vi "asdasd.vi"() -> ()   [LabVIEW 2018]
uses:
  <vilib>/userdefined/High Color/IMAQdx.ctl
  <vilib>/vision/Image Controls.llb/IMAQ Image.ctl
  <vilib>/vision/driver/NI_Vision_Acquisition_Software.lvlib
  <resource>/objmgr/imaqdx.rc
panel:
  in  "VideoMode":u32
  out "Image":T1(plugin-control)
  out "selected path":path caption="선택된 경로"
  out "Image Out":T1
  in  "Session In":T2
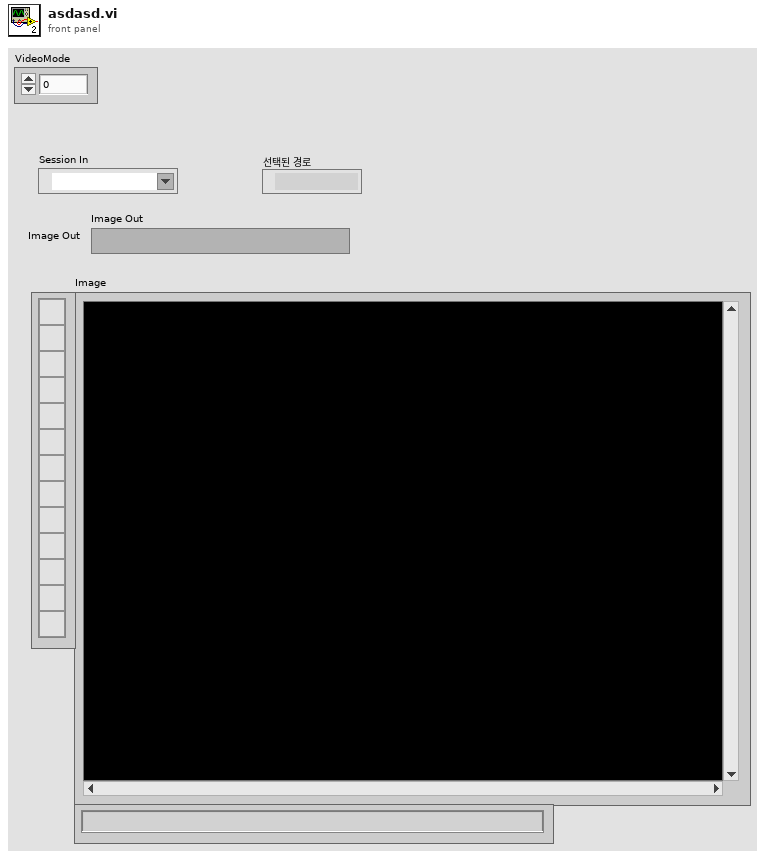
[diagram p1: front panel]
types:
  T1 = typedef "IMAQ Image.ctl" = refnum<image>
  T2 = typedef "IMAQdx.ctl" = refnum<k21>
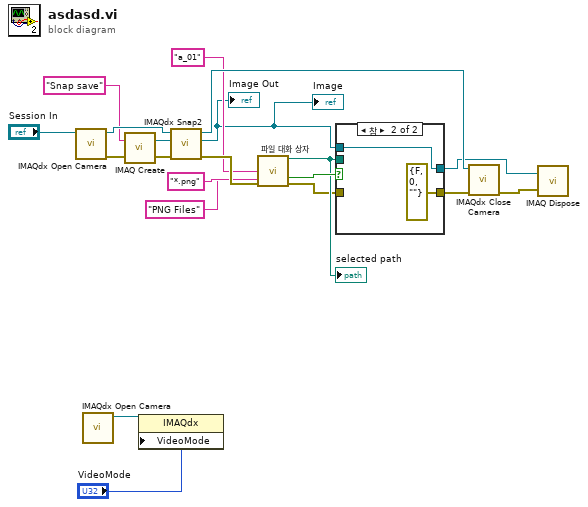
[diagram p0: block diagram]
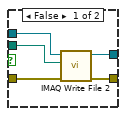
[diagram p2: hidden frame]
diagram:
  n1 = call <vilib>:"IMAQdx Open Camera.vi"("Session In"="Session In") -> ("error out"=w19:errorcluster, "Session Out"=w20:T2)  [unwired: 9 in]
  n2 = call <vilib>:"IMAQdx Open Camera.vi"() -> ("Session Out"=w2:T2)  [unwired: 10 in, 1 out]
  n3 = call "IMAQ Create"("Image Name"="Snap save", "error in (no error)"=w19) -> ("New Image"=w15:T1, "error out"=w18:errorcluster)  [unwired: 3 in]
  n4 = property class="IMAQdx"(reference=w2, "VideoMode"="VideoMode") -> ()  [unwired: 1 in, 2 out]
  n5 = call <vilib>:"IMAQdx Snap2.vi"("error in"=w18, "Image In"=w15, "Session In"=w20) -> ("error out"=w12:errorcluster, "Image Out"=w3:T1, "Session Out"=w14:T2)  [unwired: 6 in]
  "Image Out" <- w3
  "Image" <- w3
  n6 = call "파일 대화 상자"("default name"="a_01", "error in"=w12, "pattern (all files)"="*.png", "pattern label"="PNG Files") -> ("selected path"=w7:path, "cancelled"=w8:bool, "error out"=w6:errorcluster)  [unwired: 8 in, 1 out]
  "selected path" <- w7
  n7 = case shown="참" w8 {
    tunnel: w3 -> [w25 w27]
    tunnel: w7 -> [w24 _]
    tunnel: w6 -> [w23 _]
    tunnel: [w22 w27] -> w5
    tunnel: [w21 errorcluster {"status"=FALSE, "code"=0, "source"=""} ("error out")] -> w4
    frame False {
      n8 = call-poly "IMAQ Write File 2"("error in (no error)"=w23, "File Path"=w24, "Image"=w25) -> ("error out"=w21:errorcluster, "Image Out (duplicate)"=w22:T1)  [unwired: 7 in]
    }
    frame True {
    }
  }
  n9 = call <vilib>:"IMAQdx Close Camera.vi"("error in"=w4, "Session In"=w14) -> ("error out"=w13:errorcluster)  [unwired: 9 in]
  n10 = call "IMAQ Dispose"("Image"=w5, "error in (no error)"=w13) -> ()  [unwired: 4 in, 1 out]
